vi "SMTP Email Open Session.vi"(5 "password":string, 6 "username":string, 7 "error in (no error)":errorcluster, 8 "timeout ms (60000)":i32=60000, 10 "mail server":string) -> (0 "error out":errorcluster, 1 "reply 3":string, 3 "smtp session out":T1)   [LabVIEW 2011, in "NewNI_SMTPEmail.lvlib"]
doc: "Opens a TCP connection to the SMTP server specified as Mailserver, and sends it a HELO command. This VI returns a \"SMTP Session out\" and results of error interpretation in the \"error out\" cluster."
uses:
  NewNI_SMTPEmail.lvlib
  SMTP Email Session.ctl
panel:
  out "reply 2":string
  out "reply":string
  in  "smtp session":T1
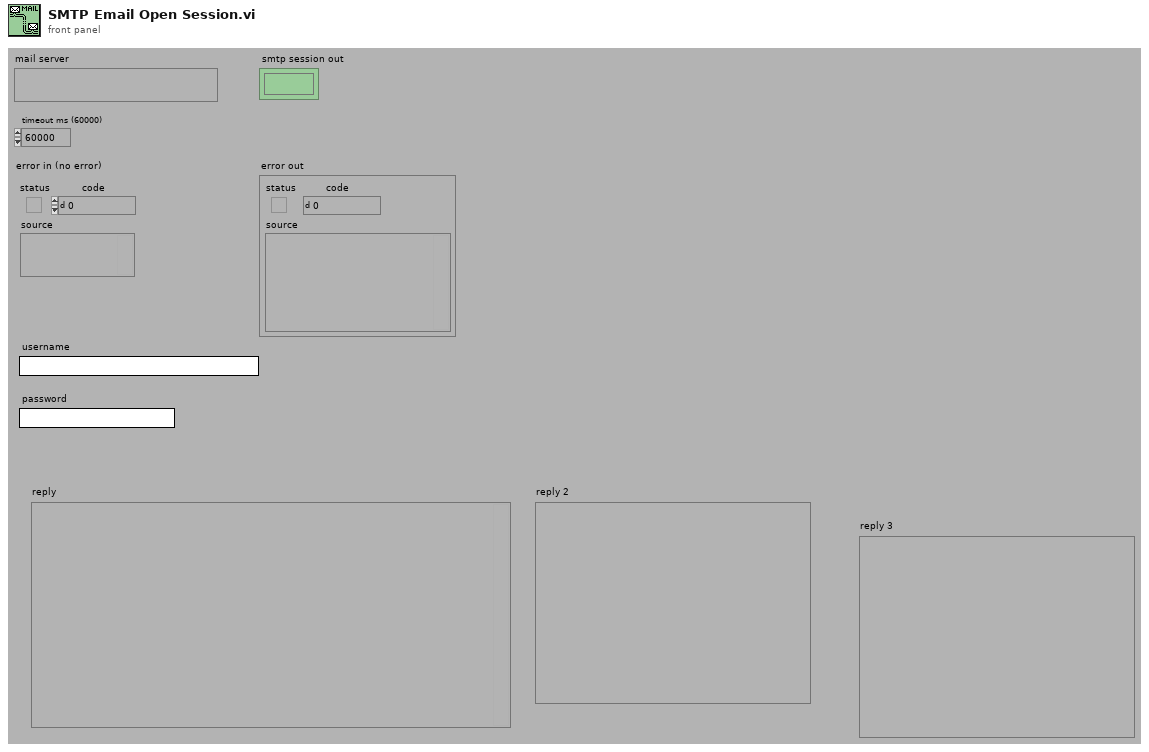
[diagram p1: front panel]
types:
  T1 = typedef "NewNI_SMTPEmail.lvlib/SMTP Email Session.ctl" = refnum<k1>
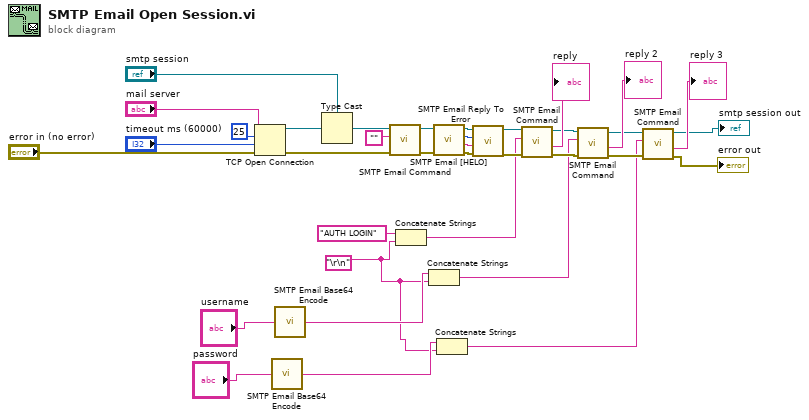
[diagram p0: block diagram]
diagram:
  w4 = "\r\n"
  n1 = TCP Open Connection(address="mail server", remote port or service name=u16 25 ("remote port"), timeout ms (60000)="timeout ms (60000)", error in (no error)="error in (no error)") -> (connection ID=w31:refnum<k5>, error out=w32:errorcluster)  [unwired: 1 out]
  n2 = call "SMTP Email Base64 Encode.vi"("Normal String"="password") -> ("Base64 String"=w5:string)  [unwired: 1 in]
  n3 = call "SMTP Email Base64 Encode.vi"("Normal String"="username") -> ("Base64 String"=w9:string)  [unwired: 1 in]
  n4 = Type Cast(type="smtp session", x=w31) -> (*(type *) &x=w34:T1)
  n5 = call "SMTP Email Command.vi"("error in (no error)"=w32, "command"="", "smtp session"=w34) -> ("error out"=w33:errorcluster, "smtp session out"=w29:T1)  [unwired: 3 out]
  n6 = Concatenate Strings("AUTH LOGIN" ("string"), w4) -> (w16:string)
  n7 = Concatenate Strings(w9, w4) -> (w10:string)
  n8 = call "SMTP Email [HELO].vi"("error in (no error)"=w33, "smtp session"=w29) -> ("error out"=w30:errorcluster, "reply"=w28:string, "reply code"=w27:i32, "smtp session out"=w26:T1)  [unwired: 1 in, 1 out]
  n9 = Concatenate Strings(w5, w4) -> (w3:string)
  n10 = call "SMTP Email Reply To Error.vi"("error in (no error)"=w30, "reply string in"=w28, "reply code in"=w27, "smtp session"=w26) -> ("error out"=w17:errorcluster, "smtp session out"=w18:T1)  [unwired: 2 out]
  n11 = call "SMTP Email Command.vi"("error in (no error)"=w17, "command"=w16, "smtp session"=w18) -> ("error out"=w12:errorcluster, "reply"=→"reply":string, "smtp session out"=w13:T1)  [unwired: 2 out]
  n12 = call "SMTP Email Command.vi"("error in (no error)"=w12, "command"=w10, "smtp session"=w13) -> ("error out"=w6:errorcluster, "reply"=→"reply 2":string, "smtp session out"=w7:T1)  [unwired: 2 out]
  n13 = call "SMTP Email Command.vi"("error in (no error)"=w6, "command"=w3, "smtp session"=w7) -> ("error out"=→"error out":errorcluster, "reply"=→"reply 3":string, "smtp session out"=→"smtp session out":T1)  [unwired: 2 out]
